vi "save binary timetrace.vi"(0 "save":bool, 1 "base path":path=path "C:/Documents and Settings/weitzlab/Desktop", 2 "raw timetrace data":u32[][](array[numeric]), 3 "Acq Rate [Hz]":dbl=100000.0 min=1.0 max=200000.0 step=1.0 format="%#_6p", 7 "filename":string="peaks_", 12 "shifts in":T1) -> (4 "save!":bool, 6 "number of files":i32, 8 "path to file":path, 14 "shifts out":T1)   [LabVIEW 2009]
uses:
  <vilib>/Utility/error.llb/DialogType.ctl
panel:
  out "?":string
  out "same file as before":bool
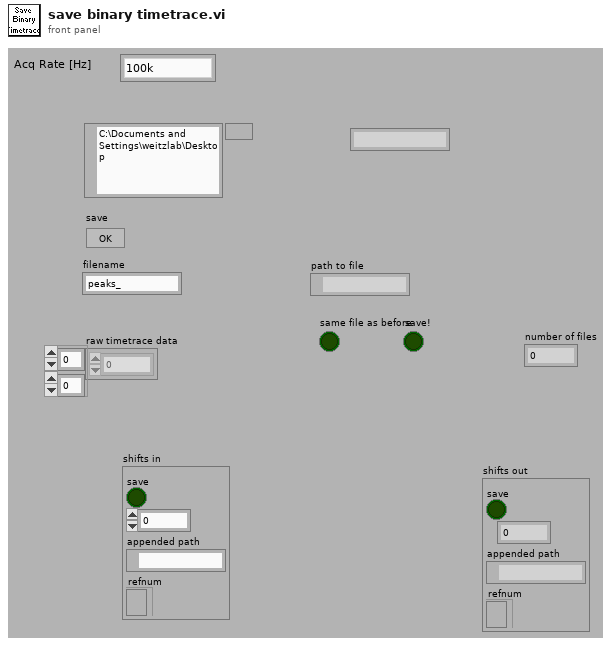
[diagram p1: front panel]
types:
  T1 = cluster{"save":bool, dbl, "appended path":path, "refnum":refnum<file>}
  T2 = enum16{"open", "replace", "create", "open or create", "replace or create", "replace or create with confirmation"}
  T3 = typedef "DialogType.ctl" = u16
  T4 = cluster{"save":bool, dbl, "appended path":path, "refnum out":refnum<file>}
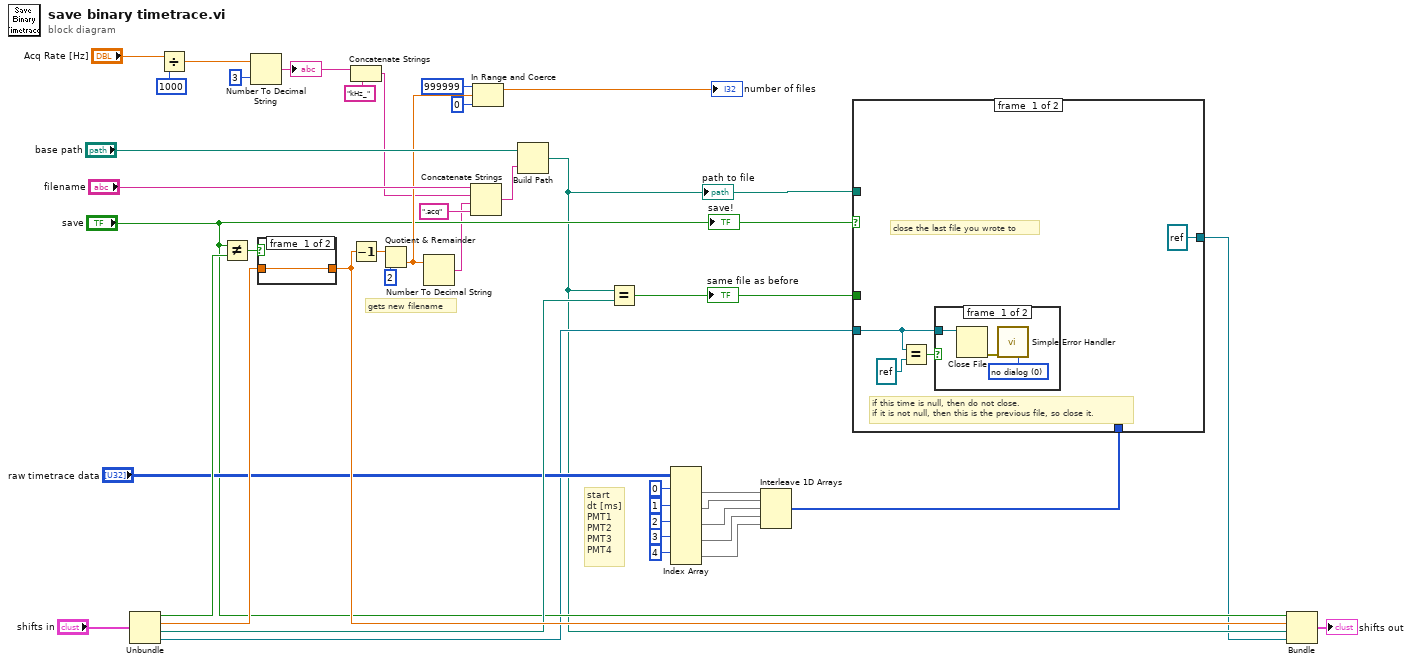
[diagram p0: block diagram]
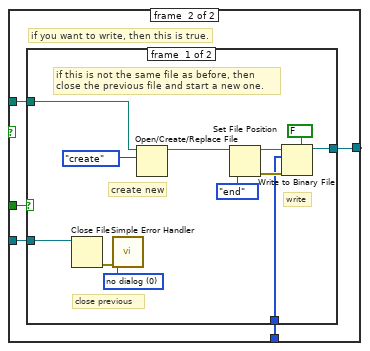
[diagram p3: hidden frame]
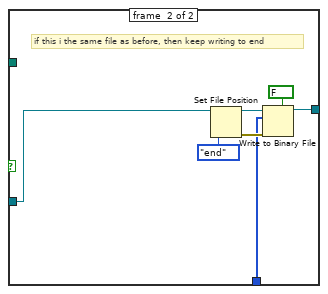
[diagram p4: hidden frame]
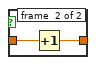
[diagram p5: hidden frame]
diagram:
  # "gets new filename"
  # "start\ndt [ms]\nPMT1\nPMT2\nPMT3\nPMT4"
  n1 = Unbundle("shifts in") -> ("save"=w36:bool, w37:dbl, "appended path"=w21:path, "refnum"=w13:refnum<file>)
  n2 = Divide(x="Acq Rate [Hz]", y=1000) -> (x/y=w5:dbl)
  n3 = Not Equal?(x="save", y=w36) -> (x != y?=w41:bool)
  n4 = Number To Decimal String(number=w5, width (-)=i16 3) -> (decimal integer string=w3:string)
  "?" <- w3
  n5 = case shown="True" w41 {
    tunnel: [w43 w45] -> w38
    tunnel: w37 -> [w43 w44]
    frame #0 {
    }
    frame #1 {
      n6 = Increment(x=w44) -> (x+1=w45:dbl)
    }
  }
  n7 = Concatenate Strings(w3, "kHz_" ("string")) -> (w1:string)
  n8 = Decrement(x=w38) -> (x-1=w39:dbl)
  n9 = Quotient & Remainder(x=w39, y=2) -> (floor(x/y)=w33:dbl)  [unwired: 1 out]
  n10 = Number To Decimal String(number=w33) -> (decimal integer string=w6:string)  [unwired: 1 in]
  n11 = Concatenate Strings("filename", w1, w6, ".acq" ("string")) -> (w34:string)
  n12 = In Range and Coerce(upper limit=999999, x=w33, lower limit=0) -> (coerced(x)=→"number of files":dbl)  [unwired: 1 out]
  n13 = Build Path(base path="base path", name or relative path=w34) -> (appended path=w12:path)
  "path to file" <- w12
  n14 = Equal?(x=w12, y=w21) -> (x = y?=w16:bool)
  "same file as before" <- w16
  n15 = Index Array(array="raw timetrace data", index (row) #1=0 ("index (row)"), index (row) #2=1 ("index (row)"), index (row) #3=2 ("index (row)"), index (row) #4=3 ("index (row)"), index (row) #5=4 ("index (row)")) -> (element #1=w25:u32[], element #2=w24:u32[], element #3=w23:u32[], element #4=w22:u32[], element #5=w18:u32[])  [unwired: 5 in]
  n16 = Interleave 1D Arrays(w25, w24, w23, w22, w18) -> (w11:u32[])
  n17 = case shown="True" "save" {
    tunnel: w16 -> [_ w57]
    tunnel: [refnum<file> refnum ("refnum out") w56] -> w10
    tunnel: w13 -> [w46 w55]
    tunnel: w12 -> [_ w54]
    tunnel: w11 -> [_ w53]
    frame #0 {
      # "if this time is null, then do not close.\nif it is not null, then this is the previous file, so close it."
      # "close the last file you wrote to"
      n18 = Equal?(x=w46, y=refnum<file> refnum ("refnum out")) -> (x = y?=w47:bool)
      n19 = case shown="False" w47 {
        tunnel: w46 -> [w51 _]
        frame #0 {
          w50 = T3 0 items=["no dialog", "OK message", "continue or stop message", "OK message + warnings", "continue/stop + warnings"] ("type of dialog (OK msg:1)")
          n20 = Close File(refnum=w51) -> (error out=w52:errorcluster)  [unwired: 1 in, 1 out]
          n21 = call <vilib>:"Simple Error Handler.vi"("type of dialog (OK msg:1)"=w50, "error in (no error)"=w52) -> ()  [unwired: 3 in, 5 out]
        }
        frame #1 {
        }
      }
    }
    frame #1 {
      # "if you want to write, then this is true."
      n22 = case shown="False" w57 {
        tunnel: [w59 w72] -> w56
        tunnel: w55 -> [w67 w71]
        tunnel: w54 -> [w65 _]
        tunnel: w53 -> [w58 w70]
        frame #0 {
          w69 = T3 0 items=["no dialog", "OK message", "continue or stop message", "OK message + warnings", "continue/stop + warnings"] ("type of dialog (OK msg:1)")
          # "write"
          # "create new"
          # "close previous"
          # "if this is not the same file as before, then close the previous file and start a new one."
          n23 = Close File(refnum=w67) -> (error out=w68:errorcluster)  [unwired: 1 in, 1 out]
          n24 = call <vilib>:"Simple Error Handler.vi"("type of dialog (OK msg:1)"=w69, "error in (no error)"=w68) -> ()  [unwired: 3 in, 5 out]
          n25 = Open/Create/Replace File(file path (use dialog)=w65, operation (0:open)=T2."create") -> (refnum out=w60:refnum<file>)  [unwired: 4 in, 2 out]
          n26 = Set File Position(refnum=w60, from (0:start)=enum16{"start", "end", "current"}."end" ("pos mode (0:2)")) -> (refnum out=w63:refnum<file>, error out=w61:errorcluster)  [unwired: 2 in]
          n27 = Write to Binary File(file (use dialog)=w63, data=w58, error in=w61, 5:FALSE ("prepend array or string size? (T)")) -> (refnum out=w59:refnum<file>)  [unwired: 2 in, 2 out]
        }
        frame #1 {
          # "if this i the same file as before, then keep writing to end"
          n28 = Set File Position(refnum=w71, from (0:start)=enum16{"start", "end", "current"}."end" ("pos mode (0:2)")) -> (refnum out=w75:refnum<file>, error out=w73:errorcluster)  [unwired: 2 in]
          n29 = Write to Binary File(file (use dialog)=w75, data=w70, error in=w73, 5:FALSE ("prepend array or string size? (T)")) -> (refnum out=w72:refnum<file>)  [unwired: 2 in, 2 out]
        }
      }
    }
  }
  n30 = Bundle("save"="save", w38, "appended path"=w12, "refnum out"=w10) -> (→"shifts out":T4)  [unwired: 1 in]
  "save!" <- "save"
